vi "PA warning message ctl.vi"(9 "get info?":bool) -> ()   [LabVIEW 2014]
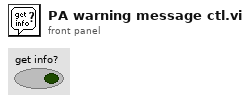
[diagram p1: front panel]
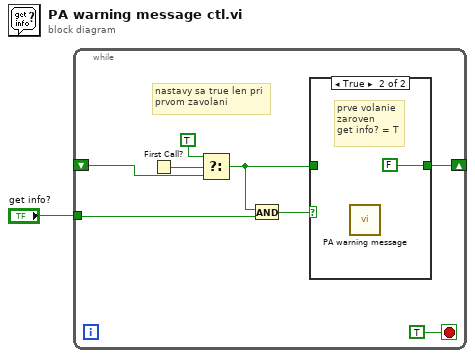
[diagram p0: block diagram]
diagram:
  n1 = while {
    shift-right: [w8] -> _
    shift-left: _ -> [w3]
    tunnel: "get info?" -> [w6]
    stop <- TRUE stop-if-true
    # "nastavy sa true len pri\nprvom zavolani"
    n2 = First Call?() -> (First Call?: T/F=w5:bool)
    n3 = Select(t=TRUE, s=w5, f=w3) -> (s? t:f=w2:bool)
    n4 = And(x=w2, y=w6) -> (x .and. y?=w7:bool)
    n5 = case shown="True" w7 {
      tunnel: [w10 FALSE] -> w8
      tunnel: w2 -> [w10 _]
      frame False {
      }
      frame True {
        # "prve volanie\nzaroven \nget info? = T"
        n6 = call "PA warning message.vi"() -> ()  [unwired: 12 in]
      }
    }
  }
